vi "NIProducts.vi"() -> ()   [LabVIEW 2015]
uses:
  <vilib>/Utility/file.llb/Read Delimited Spreadsheet (string).vi
panel:
  out "Numeric":i32
  out "subarray":string[](array[string])
  out "all rows":string[][](array[string])
  out "Key Array 4":T1(array[cluster])
  out "Key Array 3":T1(array[cluster])
  out "Key Array 2":T1(array[cluster])
  out "Key Array":T1(array[cluster])
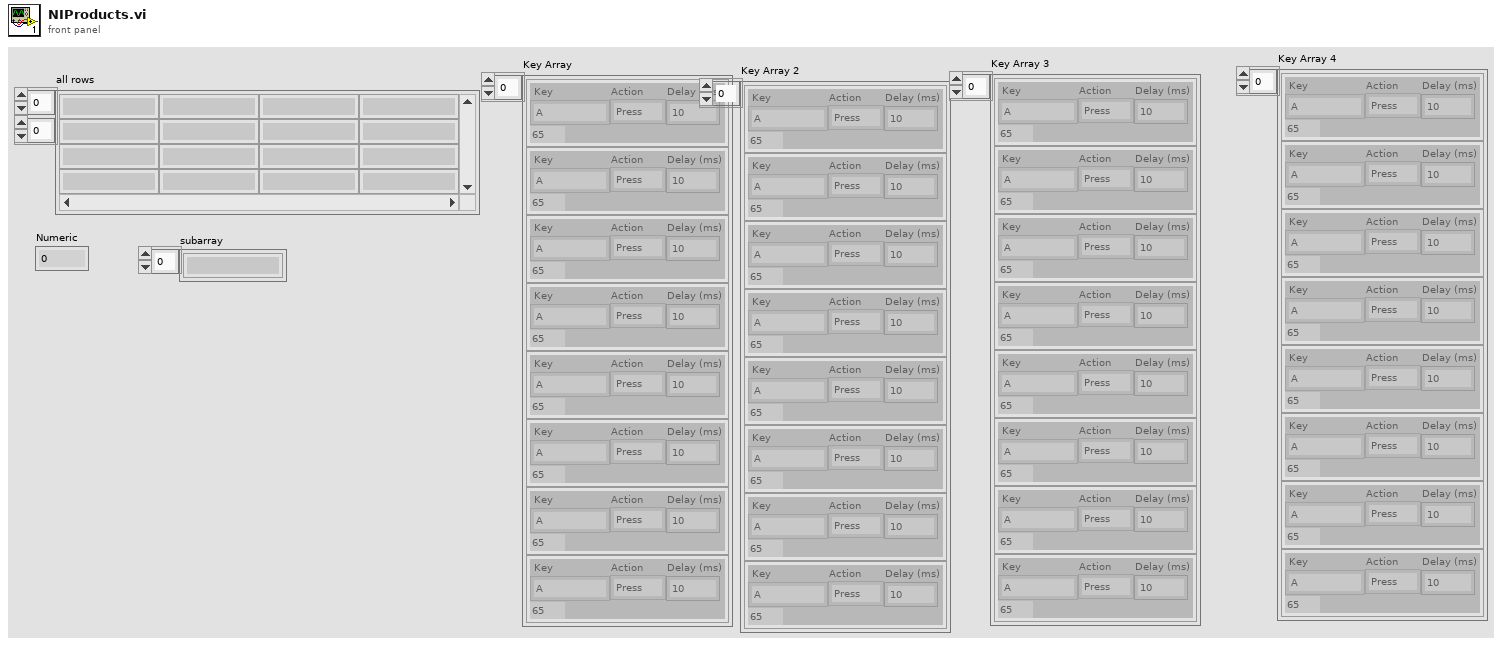
[diagram p1: front panel]
types:
  T1 = cluster{" Key":u8, "Action":enum16{"Press", "Up", "Down"}, "Delay (ms)":u32}[]
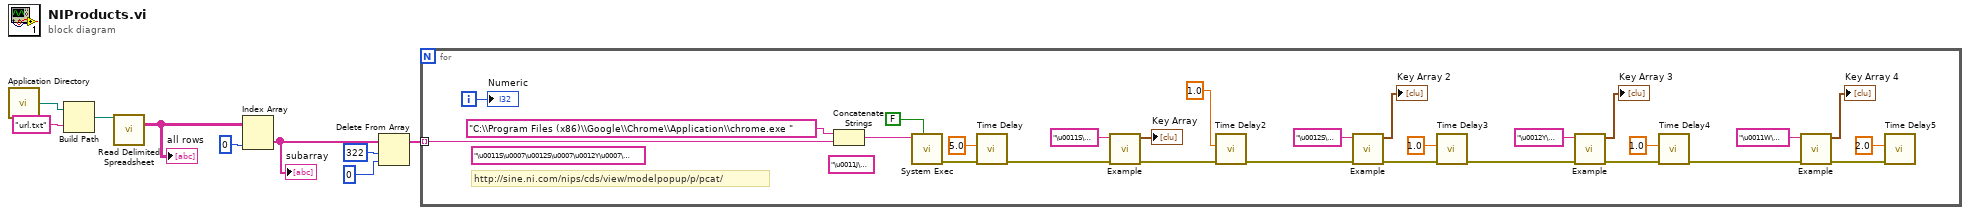
[diagram p0: block diagram]
diagram:
  n1 = call <vilib>:"Application Directory.vi"() -> ("Application Directory"=w7:path)
  n2 = Build Path(base path=w7, name or relative path="url.txt") -> (appended path=w8:path)
  n3 = call-poly <vilib>:"Read Delimited Spreadsheet.vi"("file path (dialog if empty)"=w8) -> ("all rows"=w6:string[][])  [unwired: 9 in, 5 out]
  "all rows" <- w6
  n4 = Index Array(array=w6, index (col)=0 ("disabled index (col)")) -> (element=w4:string[])  [unwired: 1 in]
  "subarray" <- w4
  n5 = Delete From Array(array=w4, length=322, index=0) -> (array with subset deleted=w3:string[])  [unwired: 1 out]
  n6 = for {
    tunnel: w3 -> [w11] mode=indexing
    i -> [w10]
    (unwired) "\u0011S\u0007\u0012S\u0007\u0012Y\u0007\u0011W\u0007" ("Input")
    (unwired) "\u0011J\u0007" ("Input")
    # "http://sine.ni.com/nips/cds/view/modelpopup/p/pcat/"
    n7 = Concatenate Strings("C:\\Program Files (x86)\\Google\\Chrome\\Application\\chrome.exe " ("command line"), w11) -> (w12:string)
    n8 = call <vilib>:"System Exec.vi"("wait until completion? (T)"=FALSE, "command line"=w12) -> ("error out"=w35:errorcluster)  [unwired: 6 in, 3 out]
    n9 = call "Time Delay"("error in (no error)"=w35, "Delay Time (s)"=5.0) -> ("error out"=w34:errorcluster)  [unwired: 9 in]
    n10 = call "Example.vi"("error in (no error)"=w34, "Input"="\u0011S\u0007") -> ("error out"=w32:errorcluster, "Key Array"=→"Key Array":T1)  [unwired: 8 in]
    n11 = call "Time Delay2"("error in (no error)"=w32, "Delay Time (s)"=1.0) -> ("error out"=w16:errorcluster)  [unwired: 9 in]
    n12 = call "Example.vi"("error in (no error)"=w16, "Input"="\u0012S\u0007") -> ("error out"=w25:errorcluster, "Key Array"=→"Key Array 2":T1)  [unwired: 8 in]
    n13 = call "Time Delay3"("error in (no error)"=w25, "Delay Time (s)"=1.0) -> ("error out"=w15:errorcluster)  [unwired: 9 in]
    n14 = call "Example.vi"("error in (no error)"=w15, "Input"="\u0012Y\u0007") -> ("error out"=w24:errorcluster, "Key Array"=→"Key Array 3":T1)  [unwired: 8 in]
    n15 = call "Time Delay4"("error in (no error)"=w24, "Delay Time (s)"=1.0) -> ("error out"=w14:errorcluster)  [unwired: 9 in]
    n16 = call "Example.vi"("error in (no error)"=w14, "Input"="\u0011W\u0007") -> ("error out"=w17:errorcluster, "Key Array"=→"Key Array 4":T1)  [unwired: 8 in]
    n17 = call "Time Delay5"("error in (no error)"=w17, "Delay Time (s)"=2.0) -> ()  [unwired: 9 in, 1 out]
    "Numeric" <- w10
  }
